vi "CIEdge.vi"(8 "error in (no error)":errorcluster, 11 "reference":refnum<k24>) -> (0 "error out":errorcluster, 1 "Edge":i32(ring) items=["Rising", "Falling"], 2 "CountDirection":i32(ring) items=["CountUp", "CountDown"], 3 "reference out":refnum<k24>, 4 "InitialCount":u32)   [LabVIEW 2009]
uses:
  C:/Program Files/National Instruments/LabVIEW 2009/vi.lib/ULx/ULx_LV.dll
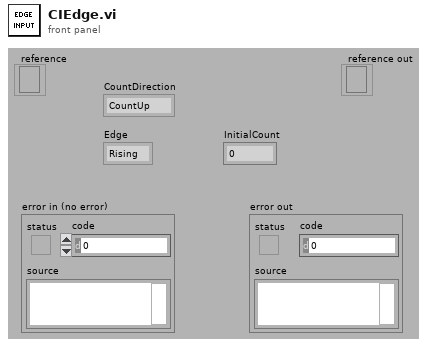
[diagram p1: front panel]
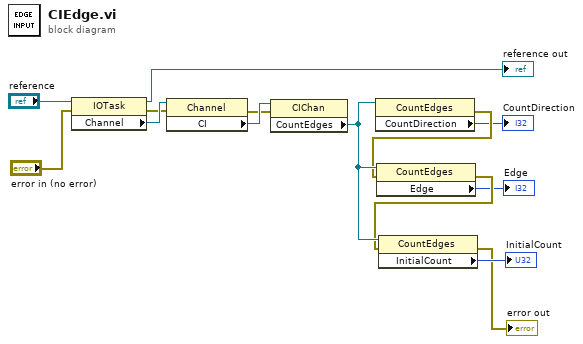
[diagram p0: block diagram]
diagram:
  n1 = property class="IOTask"(reference="reference", error in="error in (no error)") -> (reference out=→"reference out":refnum<k24>, error out=w13:errorcluster, "Channel"=w14:refnum<k24>)
  n2 = property class="Channel"(reference=w14, error in=w13) -> (error out=w10:errorcluster, "CI"=w11:refnum<k24>)  [unwired: 1 out]
  n3 = property class="CIChan"(reference=w11, error in=w10) -> ("CountEdges"=w7:refnum<k24>)  [unwired: 2 out]
  n4 = property class="CountEdges"(reference=w7) -> (error out=w6:errorcluster, "CountDirection"=→"CountDirection":i32)  [unwired: 1 in, 1 out]
  n5 = property class="CountEdges"(reference=w7, error in=w6) -> (error out=w5:errorcluster, "Edge"=→"Edge":i32)  [unwired: 1 out]
  n6 = property class="CountEdges"(reference=w7, error in=w5) -> (error out=→"error out":errorcluster, "InitialCount"=→"InitialCount":u32)  [unwired: 1 out]
